vi "GA Read Uart To Eth String.vi"(8 "error in (no error)":errorcluster caption="错误输入（无错误）", 9 "pLength":i16, 10 "pRecvBuf":string, 11 "nUartNum":i16) -> (0 "error out":errorcluster caption="错误输出", 1 "pLength out":i16, 2 "pRecvBuf out":string, 3 "function return":i32)   [LabVIEW 2015, in "GAS.lvlib"]
doc: "extern \"C\" __declspec(dllimport) int GA_ReadUartToEthString(short nUartNum,unsigned char* pRecvBuf, short* pLength);"
uses:
  <userlib>/BP_GAS/GAS.lvlib
  <userlib>/BP_GAS/GAS.dll
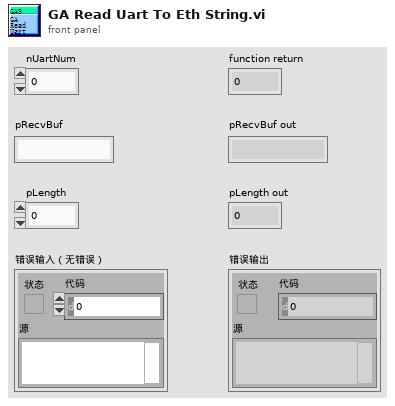
[diagram p1: front panel]
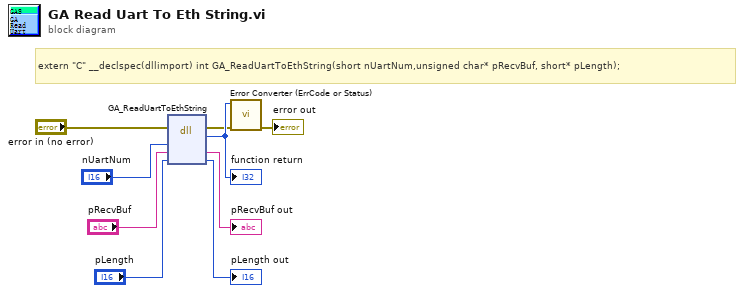
[diagram p0: block diagram]
diagram:
  # "extern \"C\" __declspec(dllimport) int GA_ReadUartToEthString(short nUartNum,unsigned char* pRecvBuf, short* pLength);"
  n1 = dll-call lib="E:/Program Files (x86)/National Instruments/LabVIEW 2015/user.lib/BP_GAS/GAS.*" fn="GA_ReadUartToEthString"(error in="error in (no error)", "nUartNum"="nUartNum", "pRecvBuf"="pRecvBuf", "pLength"="pLength") -> (error out=w2:errorcluster, w9:i32, "pRecvBuf"=→"pRecvBuf out":string, "pLength"=→"pLength out":i16)  [unwired: 3 in, 1 out]
  "function return" <- w9
  n2 = call "Error Converter (ErrCode or Status).vi"("error in (no error)"=w2, "error code"=w9) -> ("error out"=→"error out":errorcluster)  [unwired: 9 in]
